vi "MQTT ini file read write.vi"(0 "Read(F)/Write(T)?":bool, 11 "error in (no error)":errorcluster) -> (10 "Topics":string[](array[string]), 15 "error out":errorcluster)   [LabVIEW 2017]
uses:
  <vilib>/Utility/config.llb/Write Key (String).vi
  <vilib>/Utility/config.llb/NI_LVConfig.lvlib
  <vilib>/Utility/config.llb/Read Key (String).vi
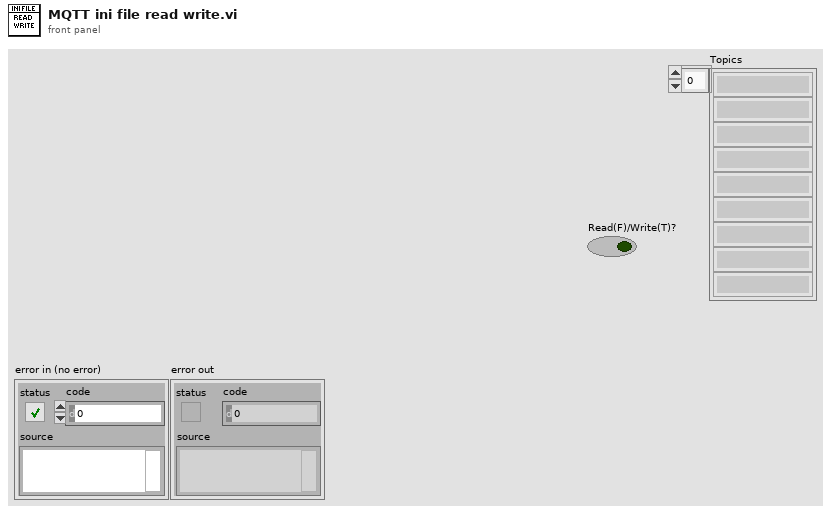
[diagram p1: front panel]
types:
  T1 = typedef "Get Path - All Path Control.ctl" = cluster{"Source Code":path, "Exe":path, "data":path, "Dynamic VI's":path, "Plugable Drivers":path, "Error Logs":path, "Database":path, "Squence":path}
  T2 = typedef "NI_LVConfig.lvlib/Config Data RefNum.ctl" = refnum<k1>
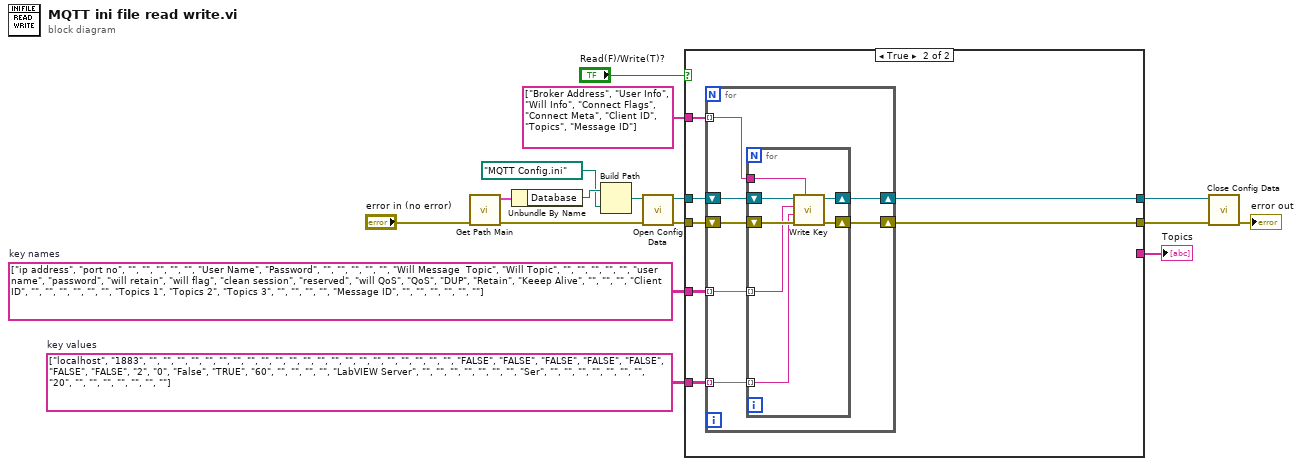
[diagram p0: block diagram]
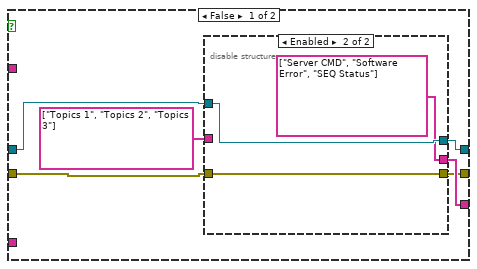
[diagram p2: hidden frame]
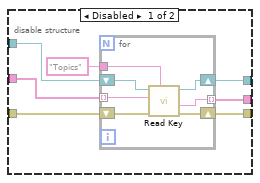
[diagram p3: hidden frame]
diagram:
  w2 = string[][] [["localhost", "1883", "", "", "", "", "", ""], ["", "", "", "", "", "", "", ""], ["", "", "", "", "", "", "", ""], ["FALSE", "FALSE", "FALSE", "FALSE", "FALSE", "FALSE", "FALSE", "2"], ["0", "False", "TRUE", "60", "", "", "", ""], ["LabVIEW Server", "", "", "", "", "", "", ""], ["Ser", "", "", "", "", "", "", ""], ["20", "", "", "", "", "", "", ""]]  # key values
  w3 = string[][] [["ip address", "port no", "", "", "", "", ""], ["User Name", "Password", "", "", "", "", ""], ["Will Message  Topic", "Will Topic", "", "", "", "", ""], ["user name", "password", "will retain", "will flag", "clean session", "reserved", "will QoS"], ["QoS", "DUP", "Retain", "Keeep Alive", "", "", ""], ["Client ID", "", "", "", "", "", ""], ["Topics 1", "Topics 2", "Topics 3", "", "", "", ""], ["Message ID", "", "", "", "", "", ""]]  # key names
  n1 = call "Get Path Main.vi"("error in (no error)"="error in (no error)") -> ("error out"=w7:errorcluster, "All Path"=w11:T1)  [unwired: 9 in]
  n2 = Unbundle By Name(w11) -> ("Database"=w10:path)
  n3 = Build Path(base path=w10, name or relative path=path "MQTT Config.ini" ("data")) -> (appended path=w8:path)
  n4 = call <vilib>:"Open Config Data.vi"("error in (no error)"=w7, "configuration file path"=w8) -> ("error out"=w15:errorcluster, "refnum"=w14:T2)  [unwired: 7 in, 1 out]
  n5 = case shown="True" "Read(F)/Write(T)?" {
    tunnel: w15 -> [w20 w44]
    tunnel: w14 -> [w17 w43]
    tunnel: [w19 w46] -> w13
    tunnel: [w18 w45] -> w12
    tunnel: string[] ["Broker Address", "User Info", "Will Info", "Connect Flags", "Connect Meta", "Client ID", "Topics", "Message ID"] ("section names") -> [_ w42]
    tunnel: w3 -> [_ w41]
    tunnel: w2 -> [_ w40]
    tunnel: [w21 _] -> w1
    frame False {
      n6 = disable-structure shown="Enabled" {
        disable-tunnel: w17 -> [w29 w39]
        disable-tunnel: w20 -> [w28 w38]
        disable-tunnel: string[] ["Topics 1", "Topics 2", "Topics 3"] ("key names") -> [w27 _]
        disable-tunnel: [w25 string[] ["Server CMD", "Software Error", "SEQ Status"]] -> w21
        disable-tunnel: [w24 w38] -> w18
        disable-tunnel: [w23 w39] -> w19
        frame Disabled {
          n7 = for {
            tunnel: "Topics" ("String") -> [w34]
            tunnel: w27 -> [w33] mode=indexing
            shift-right: [w32] -> w23
            shift-left: w29 -> [w35]
            shift-right: [w31] -> w24
            shift-left: w28 -> [w36]
            tunnel: [w30] -> w25 mode=indexing
            n8 = call-poly <vilib>:"Read Key.vi"("section"=w34, "error in (no error)"=w36, "key"=w33, "refnum"=w35) -> ("error out"=w31:errorcluster, "value"=w30:string, "refnum out"=w32:T2)  [unwired: 4 in, 1 out]
          }
        }
        frame Enabled {
        }
      }
    }
    frame True {
      n9 = for {
        shift-right: [w53] -> w46
        shift-left: w43 -> [w50]
        shift-right: [w52] -> w45
        shift-left: w44 -> [w51]
        tunnel: w42 -> [w49] mode=indexing
        tunnel: w41 -> [w48] mode=indexing
        tunnel: w40 -> [w47] mode=indexing
        n10 = for {
          tunnel: w49 -> [w58]
          tunnel: w48 -> [w57] mode=indexing
          shift-right: [w56] -> w53
          shift-left: w50 -> [w59]
          shift-right: [w55] -> w52
          shift-left: w51 -> [w60]
          tunnel: w47 -> [w54] mode=indexing
          n11 = call-poly <vilib>:"Write Key.vi"("section"=w58, "error in (no error)"=w60, "value"=w54, "key"=w57, "refnum"=w59) -> ("error out"=w55:errorcluster, "refnum out"=w56:T2)  [unwired: 4 in, 1 out]
        }
      }
    }
  }
  "Topics" <- w1
  n12 = call <vilib>:"Close Config Data.vi"("error in (no error)"=w12, "refnum"=w13) -> ("error out"=→"error out":errorcluster)  [unwired: 8 in, 1 out]
